vi "HEWH_Laurel_WaterFlowMeter.vi"(8 "error in":errorcluster, 11 "Message Queues out":T2) -> (0 "error out":errorcluster)   [LabVIEW 2023]
uses:
  Tenney/support/Message Queue/All Message Queues.ctl
  Tenney/support/Message Queue/Message Cluster.ctl
  Drivers/Laurel Meter/Type Definitions/Laurel Meter Data.ctl
  Drivers/Laurel Meter/Type Definitions/Laurel Serial Commands.ctl
  FVIR and LDO/support/Message Queue/Enqueue Message (Single).vi
  FVIR and LDO/support/Message Queue/Message Queue.lvlib
  Tenney/support/Message Queue/Tenney Message Queue.lvlib
panel:
  out "Loop Count":i32
  out "TCP Network Connection out":refnum<k5>
  out "Laurel Flow Data":T1
  in  "Debug":bool
  out "Debug":string[](array[string])
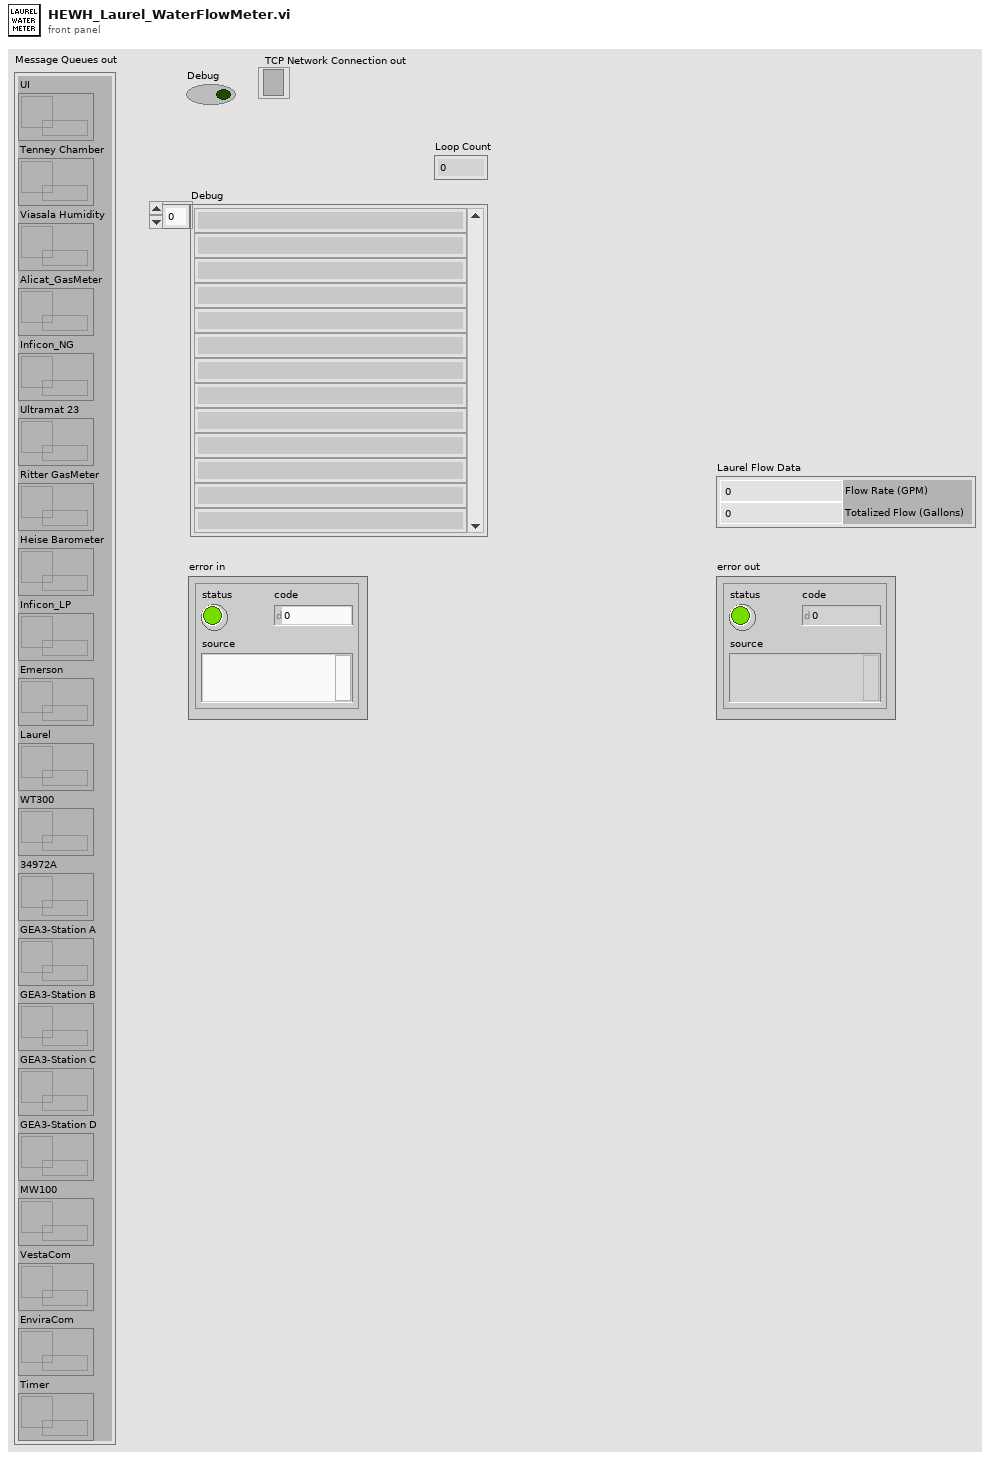
[diagram p1: front panel]
types:
  T1 = typedef "Laurel Meter Data.ctl" = cluster{"Flow Rate (GPM)":dbl, "Totalized Flow (Gallons)":dbl}
  T2 = typedef "Tenney Message Queue.lvlib/All Message Queues.ctl" = cluster{"UI":refnum<queue>, "Tenney Chamber":refnum<queue>, "Viasala Humidity":refnum<queue>, "Alicat_GasMeter":refnum<queue>, "Inficon_NG":refnum<queue>, "Ultramat 23":refnum<queue>, "Ritter GasMeter":refnum<queue>, "Heise Barometer":refnum<queue>, "Inficon_LP":refnum<queue>, "Emerson":refnum<queue>, "Laurel":refnum<queue>, "WT300":refnum<queue>, "34972A":refnum<queue>, "GEA3-Station A":refnum<queue>, "GEA3-Station B":refnum<queue>, "GEA3-Station C":refnum<queue>, "GEA3-Station D":refnum<queue>, "MW100":refnum<queue>, "VestaCom":refnum<queue>, "EnviraCom":refnum<queue>, "Timer":refnum<queue>}
  T3 = typedef "Laurel Serial Commands.ctl" = string
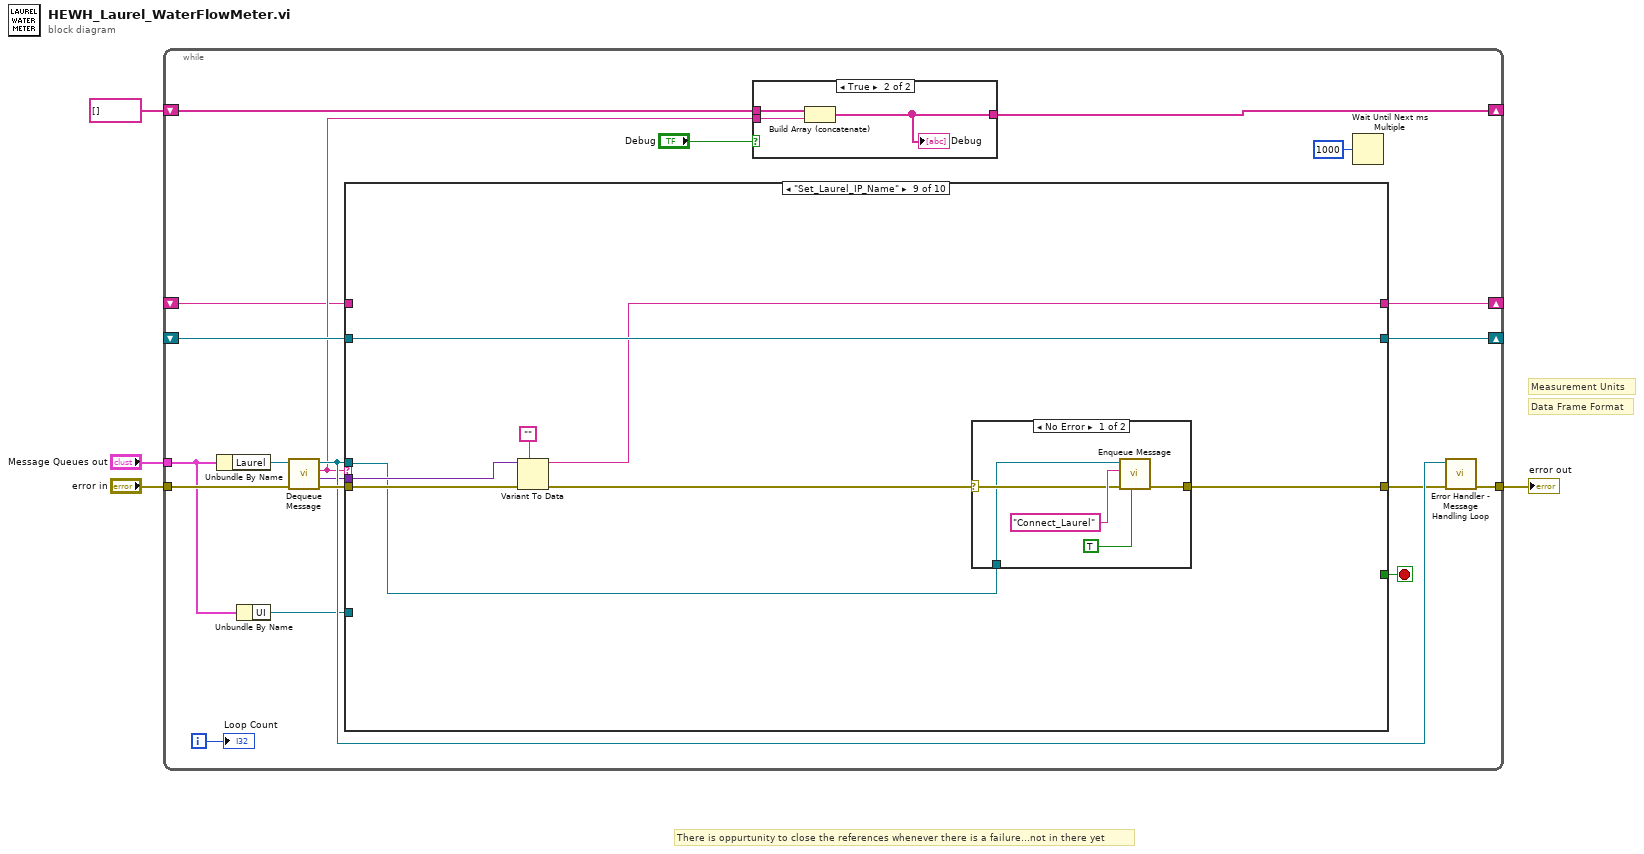
[diagram p0: block diagram]
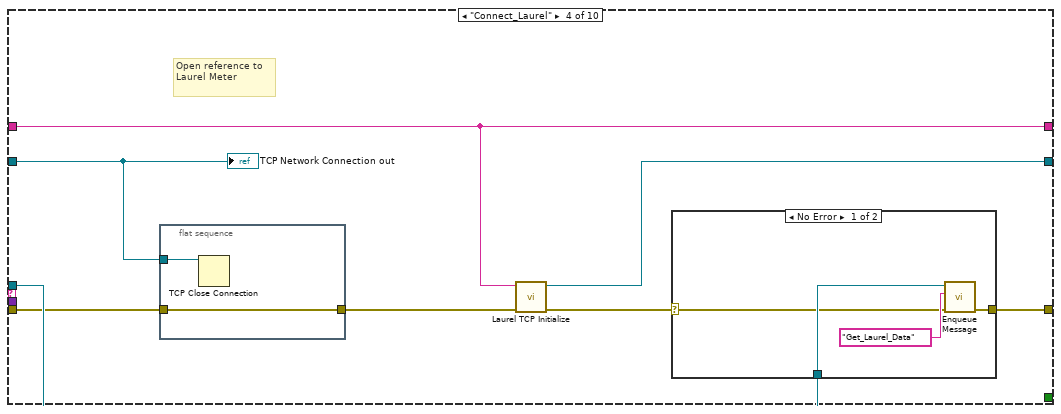
[diagram p6: hidden frame]
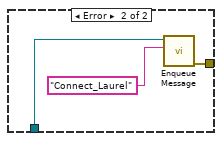
[diagram p7: hidden frame]
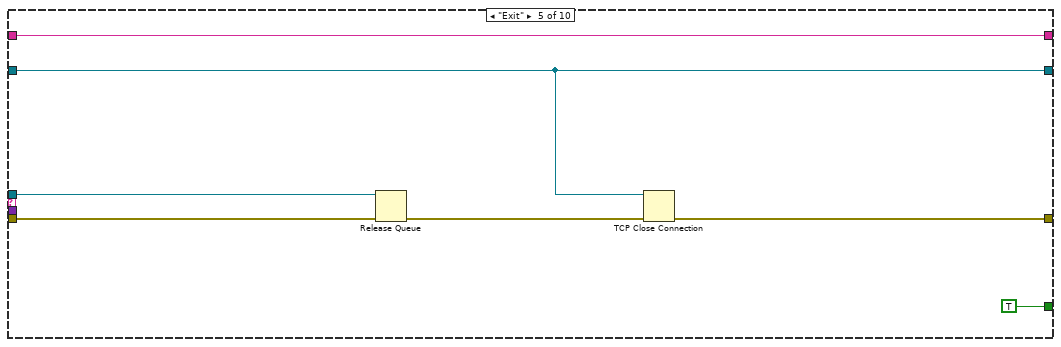
[diagram p8: hidden frame]
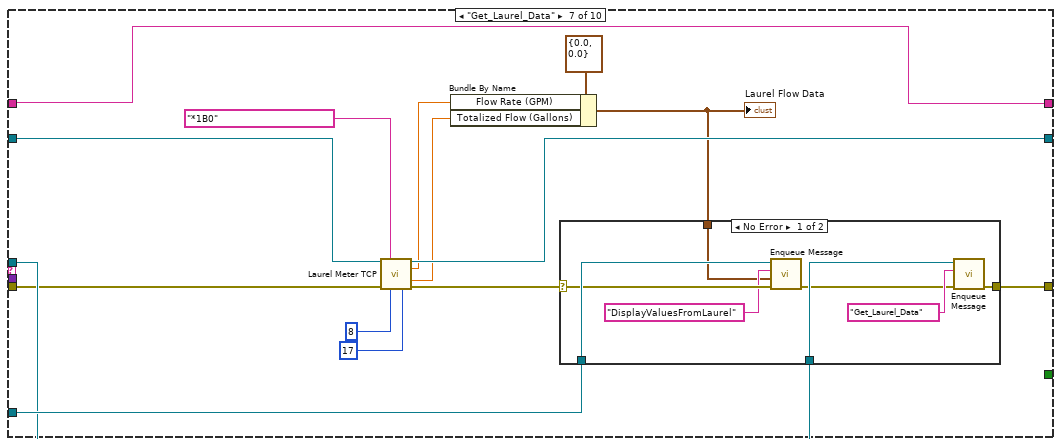
[diagram p10: hidden frame]
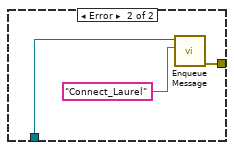
[diagram p11: hidden frame]
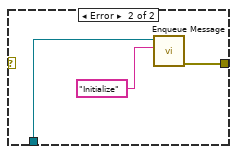
[diagram p13: hidden frame]
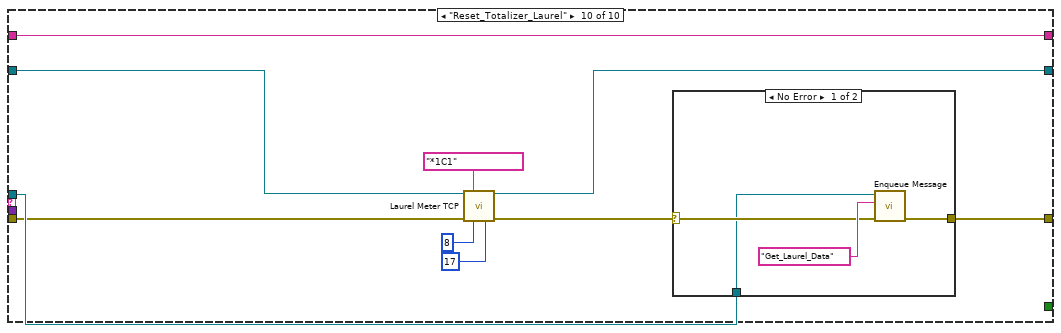
[diagram p14: hidden frame]
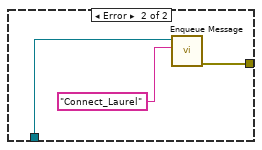
[diagram p15: hidden frame]
diagram:
  # "There is oppurtunity to close the references whenever there is a failure...not in there yet"
  # "Data Frame Format"
  # "Measurement Units"
  n1 = while {
    tunnel: "Message Queues out" -> [w14]
    tunnel: "error in" -> [w23]
    tunnel: [w19] -> w3
    shift-right: [w17] -> _
    shift-left: _ -> [w16]
    shift-right: [w10] -> _
    shift-left: string[] [] -> [w11]
    shift-right: [w7] -> _
    shift-left: _ -> [w6]
    i -> [w5]
    stop <- w21 stop-if-true
    n2 = Unbundle By Name(w14) -> ("Laurel"=w24:refnum<queue>)
    n3 = Unbundle By Name(w14) -> ("UI"=w13:refnum<queue>)
    n4 = call "Dequeue Message.vi"("error in (no error)"=w23, "Message Queue"=w24) -> ("error out"=w22:errorcluster, "Message Data"=w8:variant, "Message"=w12:string, "dup Message Queue"=w20:refnum<queue>)  [unwired: 6 in]
    n5 = case shown="\"Set_Laurel_IP_Name\"" w12 {
      tunnel: w22 -> [w30 w33 w36 w40 w59 w63 w66 w92 w99 w115]
      tunnel: [w30 w33 w36 w45 w57 w63 w78 w92 w98 w119] -> w18
      tunnel: [_ _ _ _ TRUE _ _ _ _ _] -> w21
      tunnel: w20 -> [_ _ _ w44 w60 _ w77 _ w94 w118]
      tunnel: [w31 w34 w37 w42 w56 w64 w74 w93 w101 w117] -> w17
      tunnel: w16 -> [w31 w34 w37 w38 w56 w64 w75 w93 w101 w116]
      tunnel: w13 -> [_ _ _ _ _ _ w79 _ _ _]
      tunnel: w8 -> [_ _ _ _ _ _ _ _ w97 _]
      tunnel: [w29 w32 w35 w41 w55 w62 w65 w91 w95 w110] -> w7
      tunnel: w6 -> [w29 w32 w35 w41 w55 w62 w65 w91 _ w110]
      frame "---------- Setup ----------" {
      }
      frame Default {
      }
      frame "Initialize" {
      }
      frame "Connect_Laurel" {
        # "Open reference to \nLaurel Meter"
        n6 = flat-sequence {
          tunnel: w40 -> [w47]
          tunnel: [w47] -> w39
          tunnel: w38 -> [w46]
          frame #0 {
            n7 = TCP Close Connection(connection ID=w46) -> ()  [unwired: 2 in, 2 out]
          }
        }
        n8 = call "Laurel TCP Initialize.vi"("Error In"=w39, "Laurel IP Address"=w41) -> ("Error Out"=w43:errorcluster, "Laurel Ref"=w42:refnum<k5>)  [unwired: 8 in]
        n9 = case shown="No Error" w43 {
          selector: w43 -> [w48 _]
          tunnel: [w50 w53] -> w45
          tunnel: w44 -> [w49 w52]
          frame No Error {
            n10 = call-poly "Enqueue Message.vi"("error in (no error)"=w48, "Message"="Get_Laurel_Data", "Message Queue"=w49) -> ("error out"=w50:errorcluster)  [unwired: 7 in, 1 out]
          }
          frame Error {
            n11 = call-poly "Enqueue Message.vi"("Message"="Connect_Laurel", "Message Queue"=w52) -> ("error out"=w53:errorcluster)  [unwired: 8 in, 1 out]
          }
        }
        "TCP Network Connection out" <- w38
      }
      frame "Exit" {
        n12 = Release Queue(queue=w60, error in (no error)=w59) -> (error out=w58:errorcluster)  [unwired: 1 in, 2 out]
        n13 = TCP Close Connection(connection ID=w56, error in (no error)=w58) -> (error out=w57:errorcluster)  [unwired: 1 in, 1 out]
      }
      frame "---------- Data Collection ----------" {
      }
      frame "Get_Laurel_Data" {
        n14 = call "Laurel Meter TCP.vi"("TCP Network Connection in"=w75, "Laurel Serial Commands"=T3 "*1B0", "error in (no error)"=w66, "byte count (Individual)"=8 ("byte count"), "All Items Byte Count (Flow Rate)"=17 ("byte count")) -> ("TCP Network Connection out"=w74:refnum<k5>, "Flow Rate (Item 1)"=w69:dbl, "Gallons (Item 2)"=w68:dbl, "error out"=w76:errorcluster)  [unwired: 5 in, 2 out]
        n15 = Bundle By Name(cluster=T1 {"Flow Rate (GPM)"=0.0, "Totalized Flow (Gallons)"=0.0} ("Laurel Meter Data"), "Flow Rate (GPM)"=w69, "Totalized Flow (Gallons)"=w68) -> (w67:T1)
        "Laurel Flow Data" <- w67
        n16 = case shown="No Error" w76 {
          selector: w76 -> [w82 _]
          tunnel: w79 -> [w87 _]
          tunnel: [w86 w89] -> w78
          tunnel: w77 -> [w85 w88]
          tunnel: w67 -> [w80 _]
          frame No Error {
            n17 = call-poly "Enqueue Message.vi"("error in (no error)"=w82, "Message Data"=w80, "Message"="DisplayValuesFromLaurel", "Message Queue"=w87) -> ("error out"=w83:errorcluster)  [unwired: 6 in, 1 out]
            n18 = call-poly "Enqueue Message.vi"("error in (no error)"=w83, "Message"="Get_Laurel_Data", "Message Queue"=w85) -> ("error out"=w86:errorcluster)  [unwired: 7 in, 1 out]
          }
          frame Error {
            n19 = call-poly "Enqueue Message.vi"("Message"="Connect_Laurel", "Message Queue"=w88) -> ("error out"=w89:errorcluster)  [unwired: 8 in, 1 out]
          }
        }
      }
      frame "---------- Events ----------" {
      }
      frame "Set_Laurel_IP_Name" {
        n20 = Variant To Data(error in=w99, type="", Variant=w97) -> (data=w95:string, error out=w96:errorcluster)
        n21 = case shown="No Error" w96 {
          selector: w96 -> [w104 _]
          tunnel: [w103 w108] -> w98
          tunnel: w94 -> [w102 w107]
          frame No Error {
            n22 = call-poly "Enqueue Message.vi"("Priority Message? (F)"=TRUE, "error in (no error)"=w104, "Message"="Connect_Laurel", "Message Queue"=w102) -> ("error out"=w103:errorcluster)  [unwired: 6 in, 1 out]
          }
          frame Error {
            n23 = call-poly "Enqueue Message.vi"("Message"="Initialize", "Message Queue"=w107) -> ("error out"=w108:errorcluster)  [unwired: 8 in, 1 out]
          }
        }
      }
      frame "Reset_Totalizer_Laurel" {
        n24 = call "Laurel Meter TCP.vi"("TCP Network Connection in"=w116, "Laurel Serial Commands"=T3 "*1C1", "error in (no error)"=w115, "byte count (Individual)"=8, "All Items Byte Count (Flow Rate)"=17) -> ("TCP Network Connection out"=w117:refnum<k5>, "error out"=w114:errorcluster)  [unwired: 5 in, 4 out]
        n25 = case shown="No Error" w114 {
          selector: w114 -> [w122 _]
          tunnel: [w121 w125] -> w119
          tunnel: w118 -> [w120 w124]
          frame No Error {
            n26 = call-poly "Enqueue Message.vi"("error in (no error)"=w122, "Message"="Get_Laurel_Data", "Message Queue"=w120) -> ("error out"=w121:errorcluster)  [unwired: 7 in, 1 out]
          }
          frame Error {
            n27 = call-poly "Enqueue Message.vi"("Message"="Connect_Laurel", "Message Queue"=w124) -> ("error out"=w125:errorcluster)  [unwired: 8 in, 1 out]
          }
        }
      }
    }
    n28 = case shown="True" "Debug" {
      tunnel: w12 -> [_ w28]
      tunnel: w11 -> [w25 w27]
      tunnel: [w25 w26] -> w10
      frame False {
      }
      frame True {
        n29 = Build Array (concatenate)(w27, w28) -> (w26:string[])
        "Debug" <- w26
      }
    }
    n30 = Wait Until Next ms Multiple(millisecond multiple=u32 1000) -> ()  [unwired: 1 out]
    n31 = call "Error Handler - Message Handling Loop.vi"("error in (no error)"=w18, "Message Queue"=w20) -> ("dup error in"=w19:errorcluster)  [unwired: 8 in, 1 out]
    "Loop Count" <- w5
  }
  "error out" <- w3
